vi "Teleop.vi"(10 "Match Info":T1={"Autonomous Elapsed Seconds"=0.0, "TeleOp Elapsed Seconds"=0.0, "Disabled Elapsed Seconds"=0.0, "Visited Autonomous"=FALSE, "Visited TeleOp"=FALSE, "Visited Disabled"=FALSE, "Autonomous Settings"={"Autonomous Style"=enum."Independent", "VI Refnum"=refnum}}, 11 "Call Context":T2) -> ()   [LabVIEW 2013]
doc: "This VI is called for each TeleOp packet received from the DS where the robot is not disabled. It is often used to read from the joysticks and update I/O or to update setpoints for timed control loops. It should complete and return within 20 milliseconds or it may miss DS packets."
uses:
  <vilib>/Rock Robotics/WPI/DriverStation/WPI_DriverStationDerivedRobotMode.ctl
  <vilib>/Rock Robotics/WPI/DriverStation/WPI_DriverStationMatch Info.ctl
  Driver/ADXL345 I2C Axis.ctl
  Robot Global Data.vi
  Controller 1.vi
  Drive Code/Drive 4.vi
  <vilib>/Rock Robotics/WPI/RobotDrive/WPI_RobotDriveGetSetRefNum.vi
panel:
  out "Motor Currents":dbl[](graph)
  out "Battery Voltage":dbl(graph)
  out "Velocity":dbl(graph)
  out "Acceleration":dbl(graph)
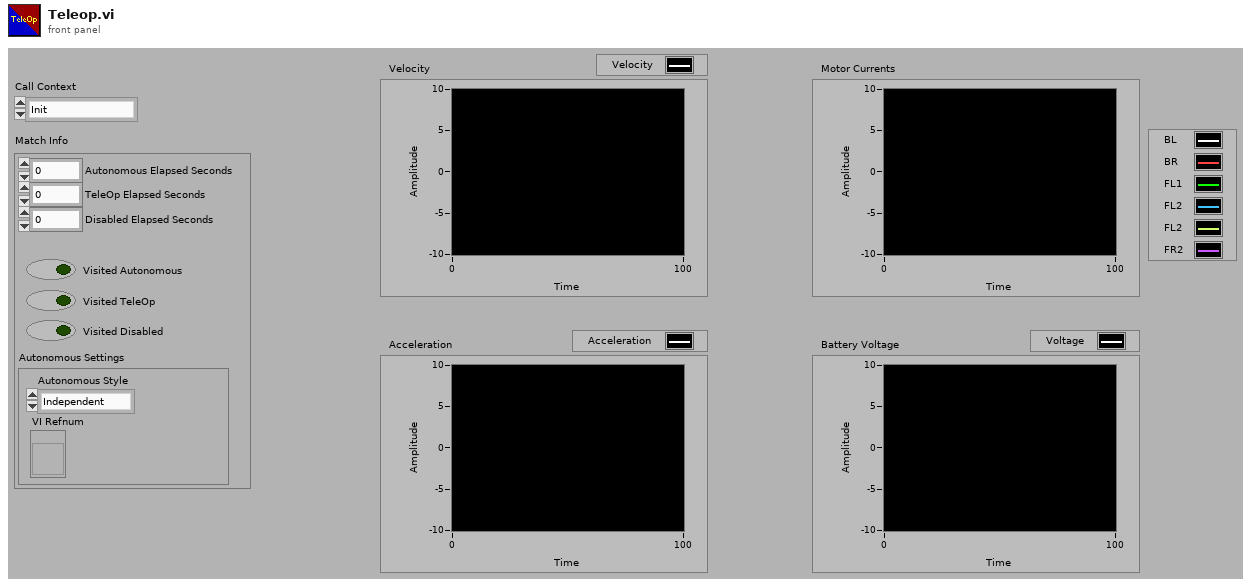
[diagram p1: front panel]
types:
  T1 = typedef "WPI_DriverStationMatch Info.ctl" = cluster{"Autonomous Elapsed Seconds":dbl, "TeleOp Elapsed Seconds":dbl, "Disabled Elapsed Seconds":dbl, "Visited Autonomous":bool, "Visited TeleOp":bool, "Visited Disabled":bool, "Autonomous Settings":cluster{"Autonomous Style":enum16{"Iterative", "Independent"}, "VI Refnum":refnum<vi>}}
  T2 = typedef "WPI_DriverStationDerivedRobotMode.ctl" = enum16{"Init", "Execute", "Stop"}
  T3 = typedef "ADXL345 I2C Axis.ctl" = u8
  T4 = cluster{"Axes":cluster{"LS X":dbl, "LS Y":dbl, "Triggers":dbl, "RS X":dbl, "RS Y":dbl}, "Buttons":cluster{"LT":bool, "RT":bool, "A":bool, "B":bool, "X":bool, "Y":bool, "LB":bool, "RB":bool, "Back":bool, "Start":bool, "LS":bool, "RS":bool}, "Buttons Just Pushed":cluster{"LT":bool, "RT":bool, "A":bool, "B":bool, "X":bool, "Y":bool, "LB":bool, "RB":bool, "Back":bool, "Start":bool, "LS":bool, "RS":bool}}
  T5 = typedef "WPI_I2CDevRef.ctl" = cluster{"DevStatus":errorcluster, "Digital Module":T6, "Device Address":u8}
  T6 = typedef "FPGA_TypedefDigitalModule.ctl" = enum16{"Digital Module 1", "Digital Module 2"}
  T7 = typedef "WPI_RobotDriveDevRef.ctl" = cluster{"DevStatus":errorcluster, "Motors[]":T8[], "Square Inputs":bool, "Max Output":dbl, "Isochronous":bool}
  T8 = typedef "WPI_MotorControlDeviceRef.ctl" = cluster{"DeviceStatus":errorcluster, "Type":enum16{"PWM", "CAN"}, "PWM":cluster{"Digital Module":T6, "PWM Channel":T9, "DeadBand":T10}, "CAN":cluster{"Device Number":u8, "Control Mode":T11, "Semaphore":T12, "Max Vout":dbl}, "Invert":bool, "TransformRef":T13, "InvTransformRef":T13}
  T9 = typedef "FPGA_DIOPWMChannel.ctl" = enum8{"PWM 1", "PWM 2", "PWM 3", "PWM 4", "PWM 5", "PWM 6", "PWM 7", "PWM 8", "PWM 9", "PWM 10", "Invalid"}
  T10 = typedef "WPI_PWMDeadband.ctl" = cluster{"Name":string, "maxPositivePwm":i32, "minPositivePwm":i32, "centerPwm":i32, "maxNegativePwm":i32, "minNegativePwm":i32, "angularRange":u16}
  T11 = typedef "WPI_CANJaguar_ControlMode.ctl" = enum8{"Percent VBus", "Current", "Speed", "Position", "Voltage"}
  T12 = typedef "Semaphore RefNum" = refnum<k1>
  T13 = typedef "WPI_PWMTransform_ConPane.ctl" = refnum<vi>
  T14 = typedef "WPI_GyroDevRef.ctl" = cluster{"DevStatus":errorcluster, "Analog Module":T15, "Analog Channel":T16, "Offset":dbl, "Gain (VoltsPerDegree/Second)":dbl}
  T15 = typedef "FPGA_TypedefAnalogModule.ctl" = enum16{"Analog Module 1", "Analog Module 2"}
  T16 = typedef "FPGA_AIChannel.ctl" = enum8{"AI 1", "AI 2", "AI 3", "AI 4", "AI 5", "AI 6", "AI 7", "AI 8", "Invalid"}
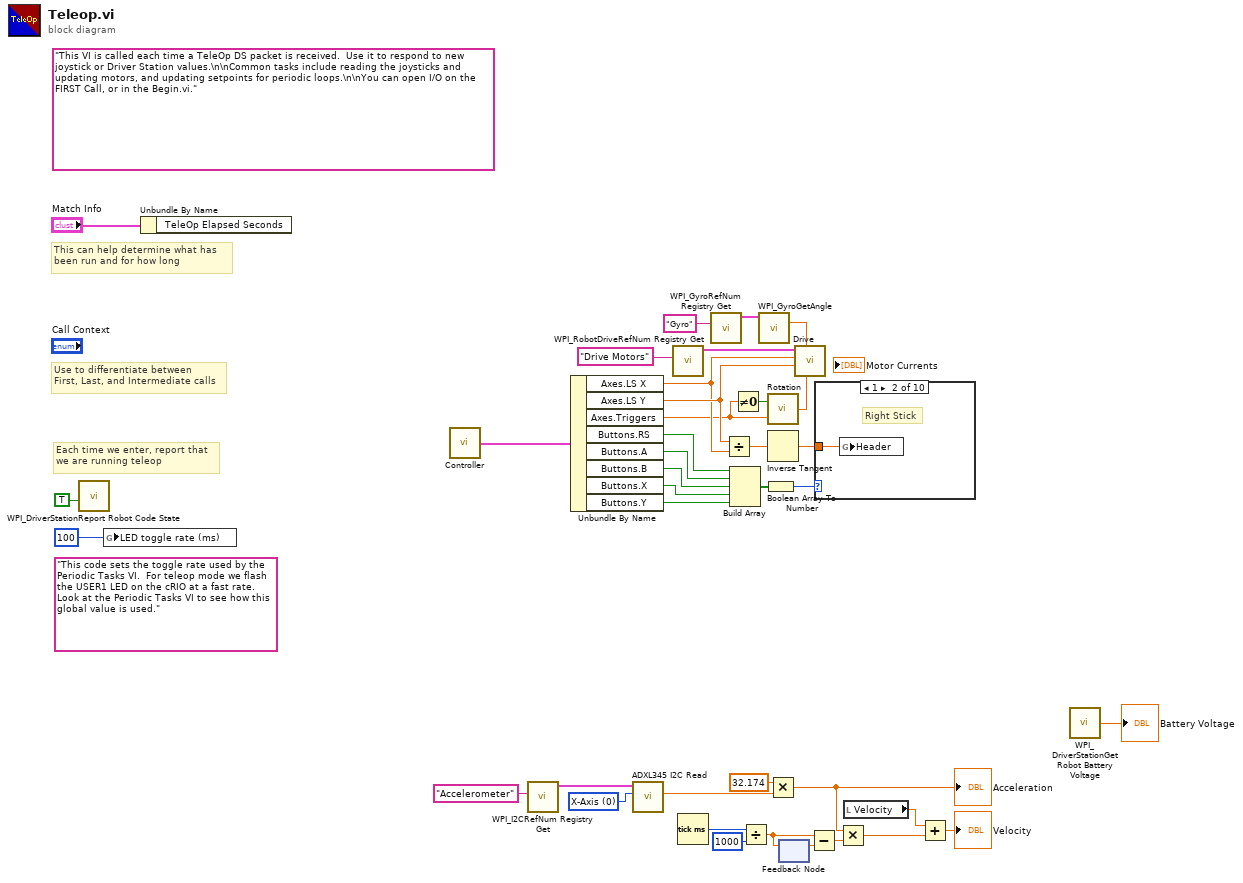
[diagram p0: block diagram]
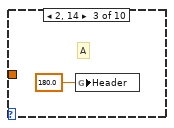
[diagram p3: hidden frame]
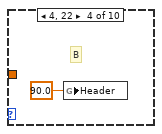
[diagram p4: hidden frame]
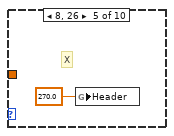
[diagram p5: hidden frame]
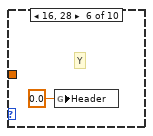
[diagram p6: hidden frame]
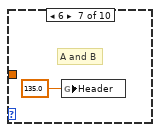
[diagram p7: hidden frame]
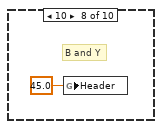
[diagram p8: hidden frame]
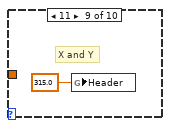
[diagram p9: hidden frame]
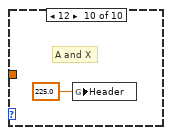
[diagram p10: hidden frame]
diagram:
  w13 = T3 0 items=["X-Axis", "Y-Axis", "Z-Axis"] ("Axis")
  (unwired) "This code sets the toggle rate used by the Periodic Tasks VI.  For teleop mode we flash the USER1 LED on the cRIO at a fast rate.  Look at the Periodic Tasks VI to see how this global value is used."
  (unwired) "This VI is called each time a TeleOp DS packet is received.  Use it to respond to new joystick or Driver Station values.\n\nCommon tasks include reading the joysticks and updating motors, and updating setpoints for periodic loops.\n\nYou can open I/O on the FIRST Call, or in the Begin.vi."
  # "Each time we enter, report that\nwe are running teleop"
  # "Use to differentiate between\nFirst, Last, and Intermediate calls"
  # "This can help determine what has\nbeen run and for how long"
  n1 = call <vilib>:"WPI_DriverStationReport Robot Code State.vi"("TeleOp"=TRUE ("Autonomous")) -> ()  [unwired: 10 in, 1 out]
  n2 = global write "Robot Global Data.vi" "LED toggle rate (ms)"(u32 100 ("LED ms toggle rate")) -> ()
  n3 = Unbundle By Name("Match Info") -> ()  [unwired: 1 out]
  n4 = call-poly "Controller.vi"() -> ("Values"=w34:T4)  [unwired: 1 in]
  n5 = call <vilib>:"WPI_I2CRefNum Registry Get.vi"("refnum name"="Accelerometer") -> ("I2CDevRef"=w14:T5)  [unwired: 9 in, 1 out]
  n6 = Unbundle By Name(w34) -> ("Axes.LS X"=w24:dbl, "Axes.LS Y"=w25:dbl, "Axes.Triggers"=w10:dbl, "Buttons.RS"=w21:bool, "Buttons.A"=w20:bool, "Buttons.B"=w19:bool, "Buttons.X"=w18:bool, "Buttons.Y"=w17:bool)
  n7 = call "ADXL345 I2C Read.vi"("Axis"=w13, "I2CDevRef"=w14) -> ("Acceleration"=w6:dbl)  [unwired: 7 in, 2 out]
  n8 = call <vilib>:"WPI_RobotDriveRefNum Registry Get.vi"("refnum name"="Drive Motors") -> ("RobotDriveDevRef"=w33:T7)  [unwired: 1 in, 9 out]
  n9 = Tick Count (ms)() -> (millisecond timer value=w9:u32)
  n10 = call <vilib>:"WPI_GyroRefNum Registry Get.vi"("refnum name"="Gyro") -> ("GyroDevRef"=w28:T14)  [unwired: 9 in, 1 out]
  n11 = Divide(x=w25, y=w24) -> (x/y=w23:dbl)
  n12 = Build Array(w21, w20, w19, w18, w17) -> (w15:bool[])
  n13 = Not Equal To 0?(x=w10) -> (x != 0?=w11:bool)
  n14 = Divide(x=w9, y=1000) -> (x/y=w2:dbl)
  n15 = call <vilib>:"WPI_GyroGetAngle.vi"("GyroDevRef"=w28) -> ("Angle"=w27:dbl)  [unwired: 7 in, 3 out]
  n16 = Boolean Array To Number(Boolean array=w15) -> (number=w16:u32)
  n17 = call "Rotation.vi"("Uncorrected Speed"=w10, "Move to Header"=w11) -> ("Output Speed"=w29:dbl)
  n18 = Inverse Tangent(1:w23) -> (0:w22:dbl)
  n19 = Multiply(x=32.174, y=w6) -> (x*y=w4:dbl)
  "Acceleration" <- w4
  n20 = feedback-in #1(w2) -> ()
  n21 = feedback #1() -> (w8:dbl)  [unwired: 1 in]
  n22 = call-poly "Drive.vi"("Rotation"=w29, "Gyro Angle"=w27, "Y"=w25, "X"=w24, "RobotDriveDevRef 2"=w33) -> ()  [unwired: 4 in, 3 out]
  n23 = Subtract(x=w2, y=w8) -> (x-y=w5:dbl)
  n24 = case shown="1" w16 {
    tunnel: w22 -> [_ w39 _ _ _ _ _ _ _ _]
    frame 0, Default {
    }
    frame 1 {
      # "Right Stick"
      n25 = global write "Robot Global Data.vi" "Header"(w39) -> ()
    }
    frame 2, 14 {
      # "A"
      n26 = global write "Robot Global Data.vi" "Header"(180.0) -> ()
    }
    frame 4, 22 {
      # "B"
      n27 = global write "Robot Global Data.vi" "Header"(90.0) -> ()
    }
    frame 8, 26 {
      # "X"
      n28 = global write "Robot Global Data.vi" "Header"(270.0) -> ()
    }
    frame 16, 28 {
      # "Y"
      n29 = global write "Robot Global Data.vi" "Header"(0.0) -> ()
    }
    frame 6 {
      # "A and B"
      n30 = global write "Robot Global Data.vi" "Header"(135.0) -> ()
    }
    frame 10 {
      # "B and Y"
      n31 = global write "Robot Global Data.vi" "Header"(45.0) -> ()
    }
    frame 11 {
      # "X and Y"
      n32 = global write "Robot Global Data.vi" "Header"(315.0) -> ()
    }
    frame 12 {
      # "A and X"
      n33 = global write "Robot Global Data.vi" "Header"(225.0) -> ()
    }
  }
  n34 = Multiply(x=w4, y=w5) -> (x*y=w3:dbl)
  n35 = local read "Velocity"() -> (w32:dbl)
  n36 = Add(x=w32, y=w3) -> (x+y=→"Velocity":dbl)
  n37 = call <vilib>:"WPI_DriverStationGet Robot Battery Voltage.vi"() -> ("robot battery voltage"=→"Battery Voltage":dbl)  [unwired: 14 in, 1 out]
